vi "Run VI.vi"(6 "Machine Name":string, 7 "Target LV Version #":T1, 8 "error in (no error)":errorcluster, 11 "VI Name":string="Client with Signaling") -> (0 "error out":errorcluster)   [LabVIEW 2025]
doc: "Author: Scott Hannahs <sth@magnet.fsu.edu>\n\nThis software is licensed for use under the “MIT License\"\nCopyright (c) 2025 Scott Hannahs, sth@sth@magnet.sthnet.net\n\nPermission is hereby granted, free of charge, to any person obtaining a copy of this software and associated documentation files (the \"Software\"), to deal in the Software without restriction, including without limitation the rights to use, copy, modify, merge, publish, distribute, sublicense, and/or sell copies of the Software, and to permit persons to whom the Software is furnished to do so, subject to the following conditions: The above copyright notice and this permission notice shall be included in all copies or substantial portions of the Software.\n\nTHE SOFTWARE IS PROVIDED \"AS IS\", WITHOUT WARRANTY OF ANY KIND, EXPRESS OR IMPLIED, INCLUDING BUT NOT LIMITED TO THE WARRANTIES OF MERCHANTABILITY, FITNESS FOR A PARTICULAR PURPOSE AND NONINFRINGEMENT. IN NO EVENT SHALL THE AUTHORS OR COPYRIGHT HOLDERS BE LIABLE FOR ANY CLAIM, DAMAGES OR OTHER LIABILITY, WHETHER IN AN ACTION OF CONTRACT, TORT OR OTHERWISE, ARISING FROM, OUT OF OR IN CONNECTION WITH THE SOFTWARE OR THE USE OR OTHER DEALINGS IN THE SOFTWARE."
uses:
  Sub Controls/LV Versions Enum.ctl
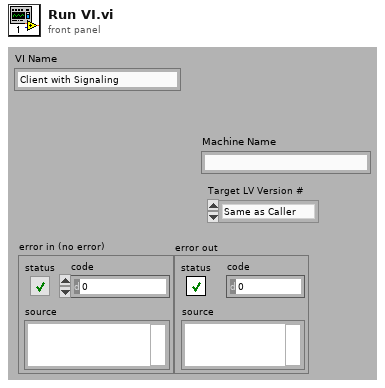
[diagram p1: front panel]
types:
  T1 = typedef "LV Versions Enum.ctl" = enum16{"Same as Caller", "8.0", "8.20", "8.5", "8.6", "9.0", "10.0", "11.0", "12.0", "13.0", "14.0", "15.0", "16.0", "17.0", "18.0", "19.0", "20.0", "21.0", "22.0", "23.0", "24.0", "25.0", "26.0", "27.0", "28.0", "29.0", "30.0"}
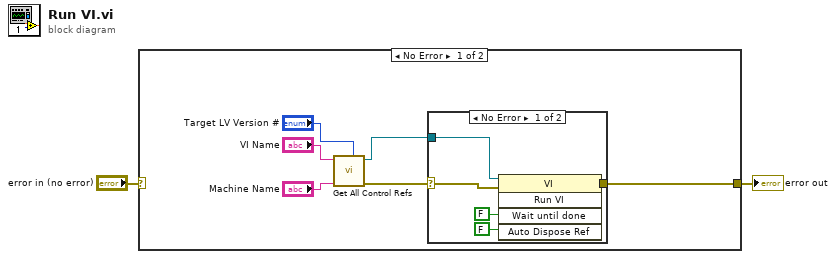
[diagram p0: block diagram]
diagram:
  n1 = case shown="No Error" "error in (no error)" {
    selector: "error in (no error)" -> [_ w15]
    tunnel: [w3 w15] -> w2
    frame No Error {
      n2 = call "Get All Control Refs.vi"("VI Name"="VI Name", "Machine Name"="Machine Name", "Target LV Version #"="Target LV Version #") -> ("VI Refnum"=w6:refnum<vi>, "error out"=w4:errorcluster)  [unwired: 3 in, 1 out]
      n3 = case shown="No Error" w4 {
        selector: w4 -> [w12 w14]
        tunnel: [w13 w14] -> w3
        tunnel: w6 -> [w11 _]
        frame No Error {
          n4 = invoke class="VI" method="Run VI"(reference=w11, error in=w12, "Wait until done"=FALSE ("Wait Until Done"), "Auto Dispose Ref"=FALSE ("Auto Dispose Reference")) -> (error out=w13:errorcluster)  [unwired: 1 in, 4 out]
        }
        frame Error {
        }
      }
    }
    frame Error {
    }
  }
  "error out" <- w2
